vi "Init Data.vi"(8 "error in":errorcluster, 9 "NumElem":i32[](array[numeric]), 10 "NumTs":i32[](array[numeric]), 11 "CRDS Data in":refnum<class "CRDS Data.lvclass">=refnum) -> (0 "error out":errorcluster, 3 "CRDS Data out":refnum<class "CRDS Data.lvclass">)   [LabVIEW 2012]
doc: "Build the arrays for the thermistor outputs, pressure transducers and the RH probes."
uses:
  Cell Class/CRDS Cell Data.lvclass
  CRDS Data.lvclass
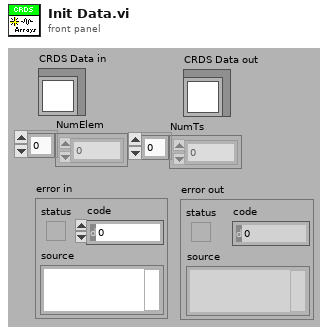
[diagram p1: front panel]
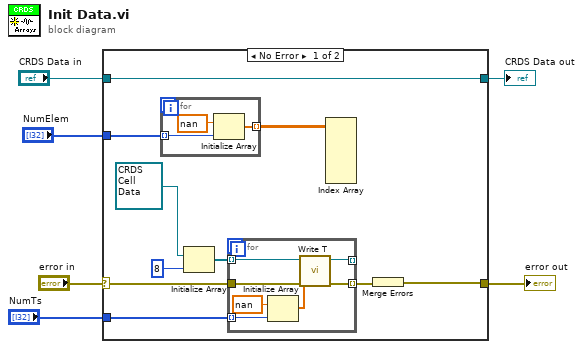
[diagram p0: block diagram]
diagram:
  n1 = case shown="No Error" "error in" {
    selector: "error in" -> [w12 w28]
    tunnel: [w9 w28] -> w5
    tunnel: [w7 w27] -> w3
    tunnel: "CRDS Data in" -> [w7 w27]
    tunnel: "NumElem" -> [w16 _]
    tunnel: "NumTs" -> [w8 _]
    frame No Error {
      n2 = for {
        tunnel: w16 -> [w26] mode=indexing
        tunnel: [w24] -> w15 mode=indexing
        n3 = Initialize Array(sgl nan ("element"), w26) -> (w24:sgl[])
      }
      n4 = Initialize Array(refnum<class "CRDS Cell Data.lvclass"> refnum ("CRDS Cell Data.lvclass"), 8 ("dimension size")) -> (w11:refnum<class "CRDS Cell Data.lvclass">[])
      n5 = for {
        tunnel: w11 -> [w23] mode=indexing
        tunnel: w8 -> [w21] mode=indexing
        tunnel: w12 -> [w19]
        tunnel: [w18] -> w10 mode=indexing
        tunnel: [w17] -> _ mode=indexing
        n6 = Initialize Array(sgl nan ("Numeric"), w21) -> (w20:sgl[])
        n7 = call-dynamic "Write T.vi"("error in"=w19, "T"=w20, "CRDS Cell Data in"=w23) -> ("error out"=w18:errorcluster, "CRDS Cell Data out"=w17:refnum<class "CRDS Cell Data.lvclass">)  [unwired: 7 in]
      }
      n8 = Index Array(array=w15) -> ()  [unwired: 6 in, 3 out]
      n9 = Merge Errors(w10) -> (w9:errorcluster)
    }
    frame Error {
    }
  }
  "error out" <- w5
  "CRDS Data out" <- w3
